vi "CallIconEditor.vi"(11 "Icon in":refnum<class "Icon.lvclass">) -> (2 "Canceled?":bool, 3 "Icon out":refnum<class "Icon.lvclass">)   [LabVIEW 2016, in "NI_NPW_Icon Overlay.lvlib"]
uses:
  <resource>/dialog/NewProjectWizard/Icon Overlay/NI_NPW_Icon Overlay.lvlib
  <vilib>/LabVIEW Icon API/lv_icon/Classes/Icon/Icon.lvclass
panel:
  out "Dummy Picture":picture
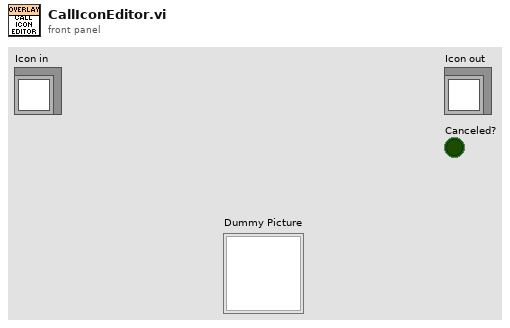
[diagram p1: front panel]
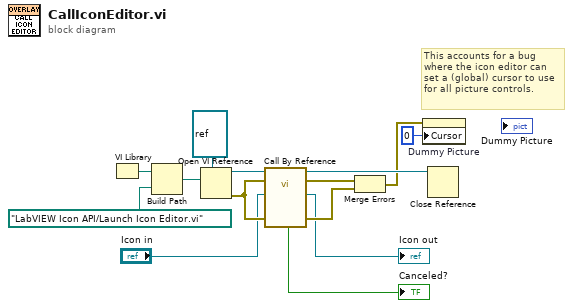
[diagram p0: block diagram]
diagram:
  # "This accounts for a bug\nwhere the icon editor can\nset a (global) cursor to use\nfor all picture controls."
  n1 = VI Library() -> (path=w11:path)
  n2 = Build Path(base path=w11, name or relative path=path "LabVIEW Icon API/Launch Icon Editor.vi" ("path")) -> (appended path=w10:path)
  n3 = Open VI Reference(type specifier VI Refnum (for type only)=refnum<vi> refnum, vi path=w10) -> (vi reference=w8:refnum<vi>, error out=w6:errorcluster)  [unwired: 4 in]
  n4 = call-by-ref "?"(reference=w8, error in=w6, 8:"error in (no error)"=w6, "Icon in"="Icon in") -> (reference out=w12:refnum<vi>, error out=w14:errorcluster, 0:"error out"=w4:errorcluster, "Icon out"=→"Icon out":refnum<class "Icon.lvclass">, "Canceled?"=→"Canceled?":bool)  [unwired: 7 in]
  n5 = Merge Errors(w14, w4) -> (w5:errorcluster)
  n6 = property on="Dummy Picture" class="Pict"(error in=w5, "Cursor"=0) -> ()  [unwired: 1 in, 2 out]
  n7 = Close Reference(reference=w12) -> ()  [unwired: 1 in, 1 out]
